vi "Init.vi"(10 "Error":errorcluster) -> (3 "Override Error Msg Strategy out":refnum<class "Override Error Msg Strategy.lvclass">)   [LabVIEW 2021, in "Override Error Msg Strategy.lvlib" / "Override Error Msg Strategy.lvclass"]
uses:
  Override Error Msg Strategy.lvclass
  Override Error Msg Strategy.lvclass/Override Error Msg Strategy.ctl
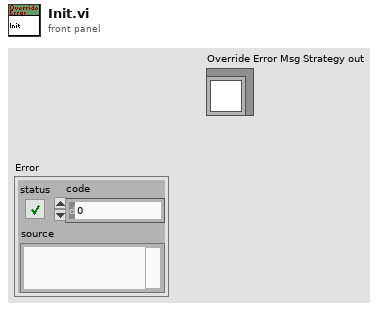
[diagram p1: front panel]
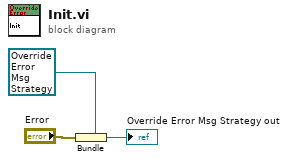
[diagram p0: block diagram]
diagram:
  n1 = Bundle(cluster=refnum<class "Override Error Msg Strategy.lvclass"> refnum ("Override Error Msg Strategy out"), "Error") -> (→"Override Error Msg Strategy out":refnum<class "Override Error Msg Strategy.lvclass">)
